vi "Process_Datatypes.vi"(8 "error in":errorcluster, 10 "dataTypes":string[](array[string]), 11 "TypeDefs":path[](array[path])) -> (0 "error out":errorcluster, 3 "final DataTypes":string[](array[string]))   [LabVIEW 2020]
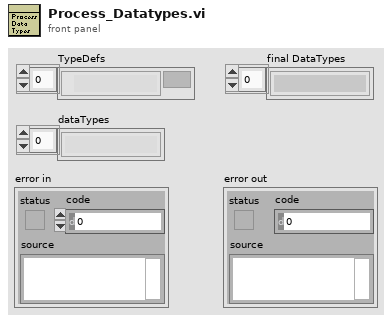
[diagram p1: front panel]
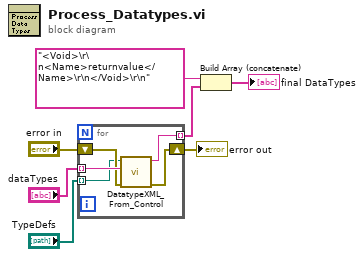
[diagram p0: block diagram]
diagram:
  n1 = for {
    tunnel: "TypeDefs" -> [w8] mode=indexing
    tunnel: "dataTypes" -> [w12] mode=indexing
    tunnel: [w11] -> w4 mode=indexing
    shift-right: [w9] -> w6
    shift-left: "error in" -> [w10]
    n2 = call <vilib>:"DatatypeXML_From_Control.vi"("error in"=w10, "Datatype"=w12, "Path"=w8) -> ("error out"=w9:errorcluster, "XML"=w11:string)  [unwired: 7 in]
  }
  "error out" <- w6
  n3 = Build Array (concatenate)("<Void>\r\n<Name>returnvalue</Name>\r\n</Void>\r\n", w4) -> (→"final DataTypes":string[])
